vi "Stop EHL (library variable).vi"() -> ()   [LabVIEW 2020, in "Error Manager.lvlib" / "New Error Dialogue GUI.lvlib"]
uses:
  New Error Dialogue GUI.lvlib
panel:
  out "Stop EHL?":bool
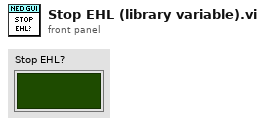
[diagram p1: front panel]
diagram:
